vi "Read Formatted Default Value.vi"(10 "# of Digits":u8=5, 11 "channel":refnum<class "TBM channel.lvclass">) -> (2 "Formatted Default":string, 3 "channel out":refnum<class "TBM channel.lvclass">)   [LabVIEW 2014, in "GraphViz Mapping Visualizer.lvlib"]
uses:
  GraphViz Mapping Visualizer.lvlib
  <vilib>/NI/Tag Bus Module Framework/channel/TBM channel.lvclass
  <vilib>/NI/Tag Bus/tag/tag descriptor.lvclass/tag descriptor.ctl
  <vilib>/NI/Tag Bus/tag/read data type.vi
  <vilib>/NI/Tag Bus/tag/tag descriptor.lvclass
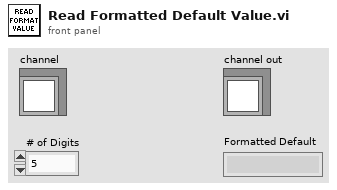
[diagram p1: front panel]
types:
  T1 = typedef "tag bus.lvlib/tag descriptor.lvclass/Data Type.ctl" = enum16{"Double", "Single", "I64", "I32", "I16", "I8", "U64", "U32", "U16", "U8", "Boolean", "String", "Array of Double", "Array of Single", "Array of I64", "Array of I32", "Array of I16", "Array of I8", "Array of U64", "Array of U32", "Array of U16", "Array of U8", "Array of Boolean", "Array of String"}
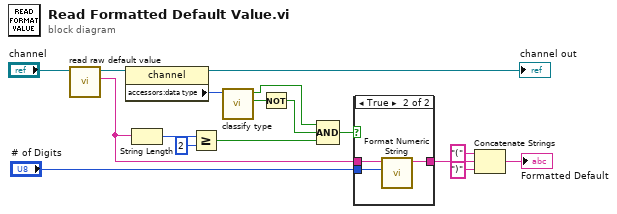
[diagram p0: block diagram]
diagram:
  n1 = call <vilib>:"read raw default value.vi"("system tag in"="channel") -> ("raw default"=w11:string, "system tag out"=w10:refnum<class "TBM channel.lvclass">)  [unwired: 8 in, 1 out]
  n2 = property class="channel"(reference=w10) -> (reference out=→"channel out":refnum<class "TBM channel.lvclass">, "accessors:data type"=w4:T1)  [unwired: 1 in, 1 out]
  n3 = String Length(string=w11) -> (length=w8:i32)
  n4 = Greater Or Equal?(x=w8, y=2) -> (x >= y?=w6:bool)
  n5 = call <vilib>:"classify type.vi"("data type"=w4) -> ("array?"=w3:bool, "numeric?"=w1:bool)  [unwired: 9 in]
  n6 = Not(x=w3) -> (.not. x?=w2:bool)
  n7 = Compound Arithmetic op=AND(w1, w2, w6) -> (w5:bool)
  n8 = case shown="True" w5 {
    tunnel: [w18 w19] -> w12
    tunnel: w11 -> [w18 w21]
    tunnel: "# of Digits" -> [_ w20]
    frame False {
    }
    frame True {
      n9 = call "Format Numeric String.vi"("digits"=w20, "default value string"=w21) -> ("formatted default value string"=w19:string)  [unwired: 9 in]
    }
  }
  n10 = Concatenate Strings("(" ("string"), w12, ")" ("string")) -> (→"Formatted Default":string)
